vi "Drive space management process.vi"() -> ()   [LabVIEW 2013]
uses:
  Global Variables/General Globals.vi
panel:
  out "Logging disabled":bool
  out "Critical Limit (GB)":dbl
  out "Below critical threshold":bool
  out "Below warning threshold":bool
  out "Warning Limit (GB)":dbl
  out "size (GB)":dbl
  out "free (GB)":dbl
  out "volume path":path
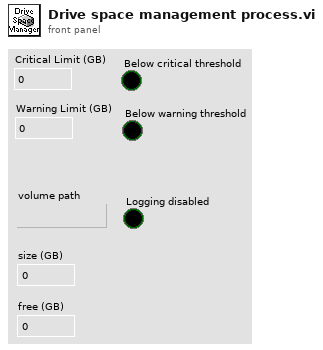
[diagram p1: front panel]
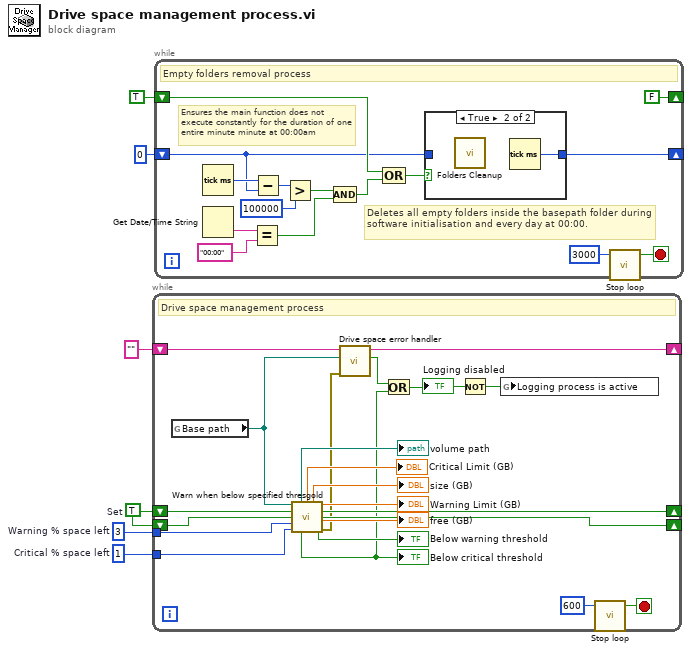
[diagram p0: block diagram]
diagram:
  w5 = TRUE  # Set
  w3 = 1  # Critical % space left
  w4 = 3  # Warning % space left
  n1 = while {
    shift-right: [w28] -> _
    shift-left: "" -> [w10]
    tunnel: w4 -> [w27]
    tunnel: w3 -> [w19]
    shift-right: [w26] -> _
    shift-left: w5 -> [w21]
    shift-right: [w17] -> _
    shift-left: w5 -> [w18]
    stop <- w7 stop-if-true
    # "Drive space management process"
    n2 = global read "General Globals.vi" "Base path"() -> (w9:path)
    n3 = call "Warn when below specified thresgold.vi"("base path"=w9, "Warning Trigger set (in)"=w21, "Critical Trigger set (in)"=w18, "Warning threshold %"=w27, "Critical threshold %"=w19) -> ("path out"=→"volume path":path, "Critical Limit (GB)"=→"Critical Limit (GB)":dbl, "size (GB)"=→"size (GB)":dbl, "Warning Limit (GB)"=→"Warning Limit (GB)":dbl, "Warning Trigger set (out)"=w26:bool, "Critical Trigger set (out)"=w17:bool, "free (GB)"=→"free (GB)":dbl, "Below critical threshold"=w14:bool, "Below warning threshold"=→"Below warning threshold":bool, "error out"=w11:errorcluster)  [unwired: 1 in]
    "Below critical threshold" <- w14
    n4 = call "Drive space error handler.vi"("error in (no error)"=w11, "Saves folder path"=w9, "String in"=w10) -> ("Boolean"=w15:bool, "String out"=w28:string)  [unwired: 7 in]
    n5 = Or(x=w15, y=w14) -> (x .or. y?=w13:bool)
    "Logging disabled" <- w13
    n6 = Not(x=w13) -> (.not. x?=w12:bool)
    n7 = global write "General Globals.vi" "Logging process is active"(w12) -> ()
    n8 = call "Stop loop.vi"("Loop iteration (ms)"=u32 600) -> ("Stop"=w7:bool)  [unwired: 4 in]
  }
  n9 = while {
    shift-right: [w39] -> _
    shift-left: u32 0 ("millisecond timer value") -> [w31]
    shift-right: [FALSE] -> _
    shift-left: TRUE -> [w37]
    stop <- w43 stop-if-true
    # "Ensures the main function does not execute constantly for the duration of one entire minute minute at 00:00am"
    # "Deletes all empty folders inside the basepath folder during software initialisation and every day at 00:00."
    # "Empty folders removal process"
    n10 = Tick Count (ms)() -> (millisecond timer value=w36:u32)
    n11 = Get Date/Time String() -> (time string=w40:string)  [unwired: 4 out]
    n12 = Equal?(x=w40, y="00:00" ("time string")) -> (x = y?=w32:bool)
    n13 = Subtract(x=w36, y=w31) -> (x-y=w35:u32)
    n14 = Greater?(x=w35, y=u32 100000) -> (0:w33:bool)
    n15 = Compound Arithmetic op=AND(w33, w32) -> (w30:bool)
    n16 = Compound Arithmetic op=OR(w37, w30) -> (w29:bool)
    n17 = case shown="True" w29 {
      tunnel: [w44 w45] -> w39
      tunnel: w31 -> [w44 _]
      frame False {
      }
      frame True {
        n18 = call "Folders Cleanup.vi"() -> ()  [unwired: 11 in, 1 out]
        n19 = Tick Count (ms)() -> (millisecond timer value=w45:u32)
      }
    }
    n20 = call "Stop loop.vi"("Loop iteration (ms)"=u32 3000) -> ("Stop"=w43:bool)  [unwired: 4 in]
  }
